vi "solar_misc Unix Time.vi"(10 "Unix Time":dbl format="%#.9f", 11 "LabVIEW Time":timestamp) -> (2 "LabVIEW Time out":timestamp, 3 "Unix Time out":dbl format="%#.9f")   [LabVIEW 2018]
doc: "This converts a LabVIEW timestamp to Unix timstamp by adjust for the Unix epoch time."
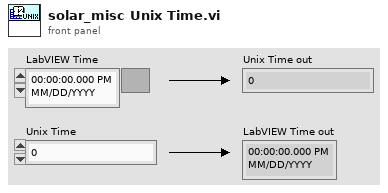
[diagram p1: front panel]
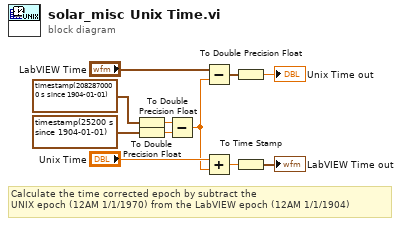
[diagram p0: block diagram]
diagram:
  # "Calculate the time corrected epoch by subtract the \nUNIX epoch (12AM 1/1/1970) from the LabVIEW epoch (12AM 1/1/1904)"
  n1 = To Double Precision Float(number=timestamp(2082870000 s since 1904-01-01)) -> (double precision float=w8:dbl)
  n2 = To Double Precision Float(number=timestamp(25200 s since 1904-01-01)) -> (double precision float=w7:dbl)
  n3 = Subtract(x=w8, y=w7) -> (x-y=w3:dbl)
  n4 = Subtract(x="LabVIEW Time", y=w3) -> (x-y=w6:timestamp)
  n5 = Add(x="Unix Time", y=w3) -> (x+y=w2:dbl)
  n6 = To Double Precision Float(number=w6) -> (double precision float=→"Unix Time out":dbl)
  n7 = To Time Stamp(1:w2) -> (0:→"LabVIEW Time out":timestamp)
